vi "test.to.str.AddOrder.1.vi"() -> ()   [LabVIEW 2020]
uses:
  fpga/orderbook.command.ctl
  fpga/orderbook.command.type.ctl
  fpganow.common.host.lvlib
  fpga/fpganow.common.fpga.lvlib
panel:
  out "match":string
  out "x = y?":bool[](array[boolean])
  out "Actual Out":string
  in  "Expected Out":string="(AddOrder, 700, ORD0001, Buy, 50 x AAPL@ 300.25)"
  out "Passed?":bool
  in  "orderbook.command":T1={"type"=enum."AddOrder", "side"=66, "orderId "=2328169985193553969, "quantity"=50, "symbol"=4702127773838221344, "price"=30025, "executed.qty"=0, "canceled.qty"=0, "remaining.qty"=0, "seconds"=44700, "nanoseconds"=700, "Add"=TRUE, "Edit"=FALSE, "Remove"=FALSE, "seq no"=0, "recv.time"=0, "parse.time"=0} {"symbol" format="%.0x"; "orderId" format="%.0x"; "side" format="%.0x"}
  # "0x42 = 'B'\n0x53 = 'S'"
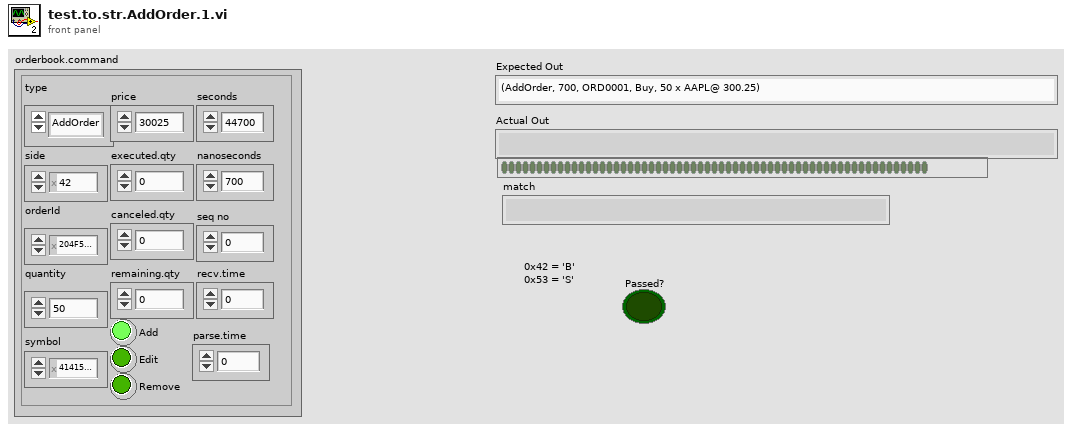
[diagram p1: front panel]
types:
  T1 = typedef "fpganow.common.fpga.lvlib/orderbook.command.ctl" = cluster{"type":T2, "side":u8, "orderId ":u64, "quantity":u32, "symbol":u64, "price":u64, "executed.qty":u32, "canceled.qty":u32, "remaining.qty":u32, "seconds":u64, "nanoseconds":u64, "Add":bool, "Edit":bool, "Remove":bool, "seq no":u32, "recv.time":u64, "parse.time":u64}
  T2 = typedef "fpganow.common.fpga.lvlib/orderbook.command.type.ctl" = enum8{"Time", "AddOrder", "OrderExecuted", "OrderExecutedAtPrice", "ReduceSize", "ModifyOrder", "DeleteOrder", "Get.Everything", "Get.All.Orders", "Get.Top"}
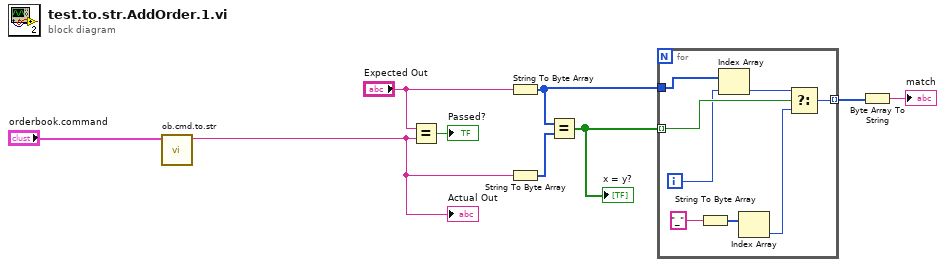
[diagram p0: block diagram]
diagram:
  n1 = call "ob.cmd.to.str.vi"("orderbook.command"="orderbook.command") -> ("string"=w6:string)  [unwired: 10 in]
  "Actual Out" <- w6
  n2 = Equal?(x="Expected Out", y=w6) -> (x = y?=→"Passed?":bool)
  n3 = String To Byte Array(string="Expected Out") -> (unsigned byte array=w4:u8[])
  n4 = String To Byte Array(string=w6) -> (unsigned byte array=w5:u8[])
  n5 = Equal?(x=w4, y=w5) -> (x = y?=w3:bool[])
  "x = y?" <- w3
  n6 = for {
    tunnel: w4 -> [w16]
    tunnel: w3 -> [w17] mode=indexing
    tunnel: [w10] -> w2 mode=indexing
    i -> [w15]
    n7 = String To Byte Array(string="_") -> (unsigned byte array=w13:u8[])
    n8 = Index Array(array=w16, index=w15) -> (element=w14:u8)
    n9 = Index Array(array=w13) -> (element=w11:u8)  [unwired: 1 in]
    n10 = Select(t=w14, s=w17, f=w11) -> (s? t:f=w10:u8)
  }
  n11 = Byte Array To String(unsigned byte array=w2) -> (string=→"match":string)
